vi "LCAIO Lookup Analog Io Device By Name.vi"(8 "error in (no error)":errorcluster caption="Fehler (Eingang, kein Fehler)", 11 "Name":string) -> (0 "error out":errorcluster caption="Fehler (Ausgang)", 3 "Analog IO Device Handle":i64)   [LabVIEW 2021, in "labbCAN_AnalogIO_API.lvlib"]
doc: "LCAIO_Func long LCAIO_CALL LCAIO_LookupAnalogIoDeviceByName(char *pName,\n dev_hdl *pAnalogIoDeviceHdl);"
uses:
  labbCAN_AnalogIO_API.lvlib
  labbCAN_AnalogIO_API.dll
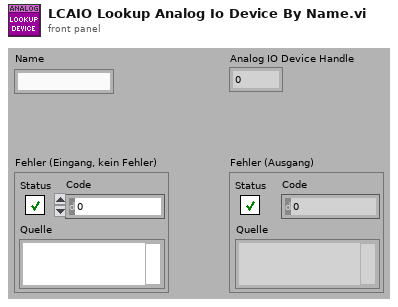
[diagram p1: front panel]
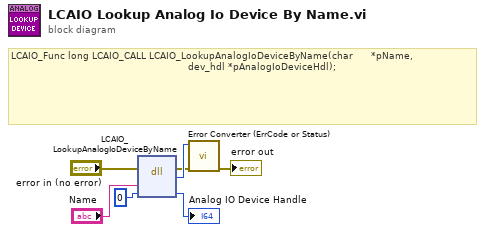
[diagram p0: block diagram]
diagram:
  # "LCAIO_Func long LCAIO_CALL LCAIO_LookupAnalogIoDeviceByName(char      *pName,\n                                                           dev_hdl *pAnalogIoDeviceHdl);"
  n1 = dll-call lib="C:/Users/olaja/AppData/Local/CETONI_SDK/labbCAN_AnalogIO_API.*" fn="LCAIO_LookupAnalogIoDeviceByName"(error in="error in (no error)", "Name"="Name", "Analog IO Device Handle"=i64 0) -> (error out=w2:errorcluster, "Rückgabetyp"=w3:i32, "Analog IO Device Handle"=→"Analog IO Device Handle":i64)  [unwired: 3 in, 1 out]
  n2 = call "Error Converter (ErrCode or Status).vi"("error in (no error)"=w2, "error code"=w3) -> ("error out"=→"error out":errorcluster)  [unwired: 9 in]
